vi "UpdateCameraSettings.vi"(10 "config":T1 {"QTrk Settings"."QI ROI Coverage" format="%_2g"; "QTrk Settings"."QI MinRadius" format="%.2f"; "QTrk Settings"."QI Angular sample density" format="%.3f"; "QTrk Settings"."QI Radial sample density" format="%.2f"; "QTrk Settings"."ZLUT Radial sample density" format="%.2f"; "QTrk Settings"."ZLUT MinRadius" format="%.2f"}, 11 "Main Camera Instance":T15) -> ()   [LabVIEW 2011]
uses:
  Main/Camera/CameraInstance.ctl
  Modules/CameraInterface/CameraInterface.ctl
  Modules/CameraInterface/CICloseType.ctl
  Modules/CameraInterface/CIGetSetGenericConfig.ctl
  Modules/CameraInterface/CIGrabType.ctl
  Modules/CameraInterface/CISettingsDlg.ctl
  Modules/CameraInterface/CIAdjustBeadPos.ctl
  Modules/CameraInterface/CISaveLoadSettings.ctl
  Main/Typedefs/MeasureConfigType.ctl
  Main/Typedefs/MeasureConfigOutputMode.ctl
  qtrk/QTrkLVBinding/QTrkSettings.ctl
  Main/Typedefs/TrackingConfigType.ctl
  qtrk/QTrkLVBinding/QTrkLocalizationType.ctl
  qtrk/QTrkLVBinding/QTrkZCommandType.ctl
  Main/ExperimentProgram/ExperimentProgramType.ctl
  Main/ExperimentProgram/ExProgCommandType.ctl
  Main/ExperimentProgram/ExProgCommandEnumType.ctl
  Main/Motors/MotorAxisEnum.ctl
  Main/Motors/MotorPosType.ctl
  Main/Typedefs/XYf.ctl
  Main/Motors/MotorPosFlagsType.ctl
  Main/Camera/GenericCameraConfigType.ctl
panel:
  # "(used for commands with string parameters)"
  # "-2: Use all devices\n-1: Use best device"
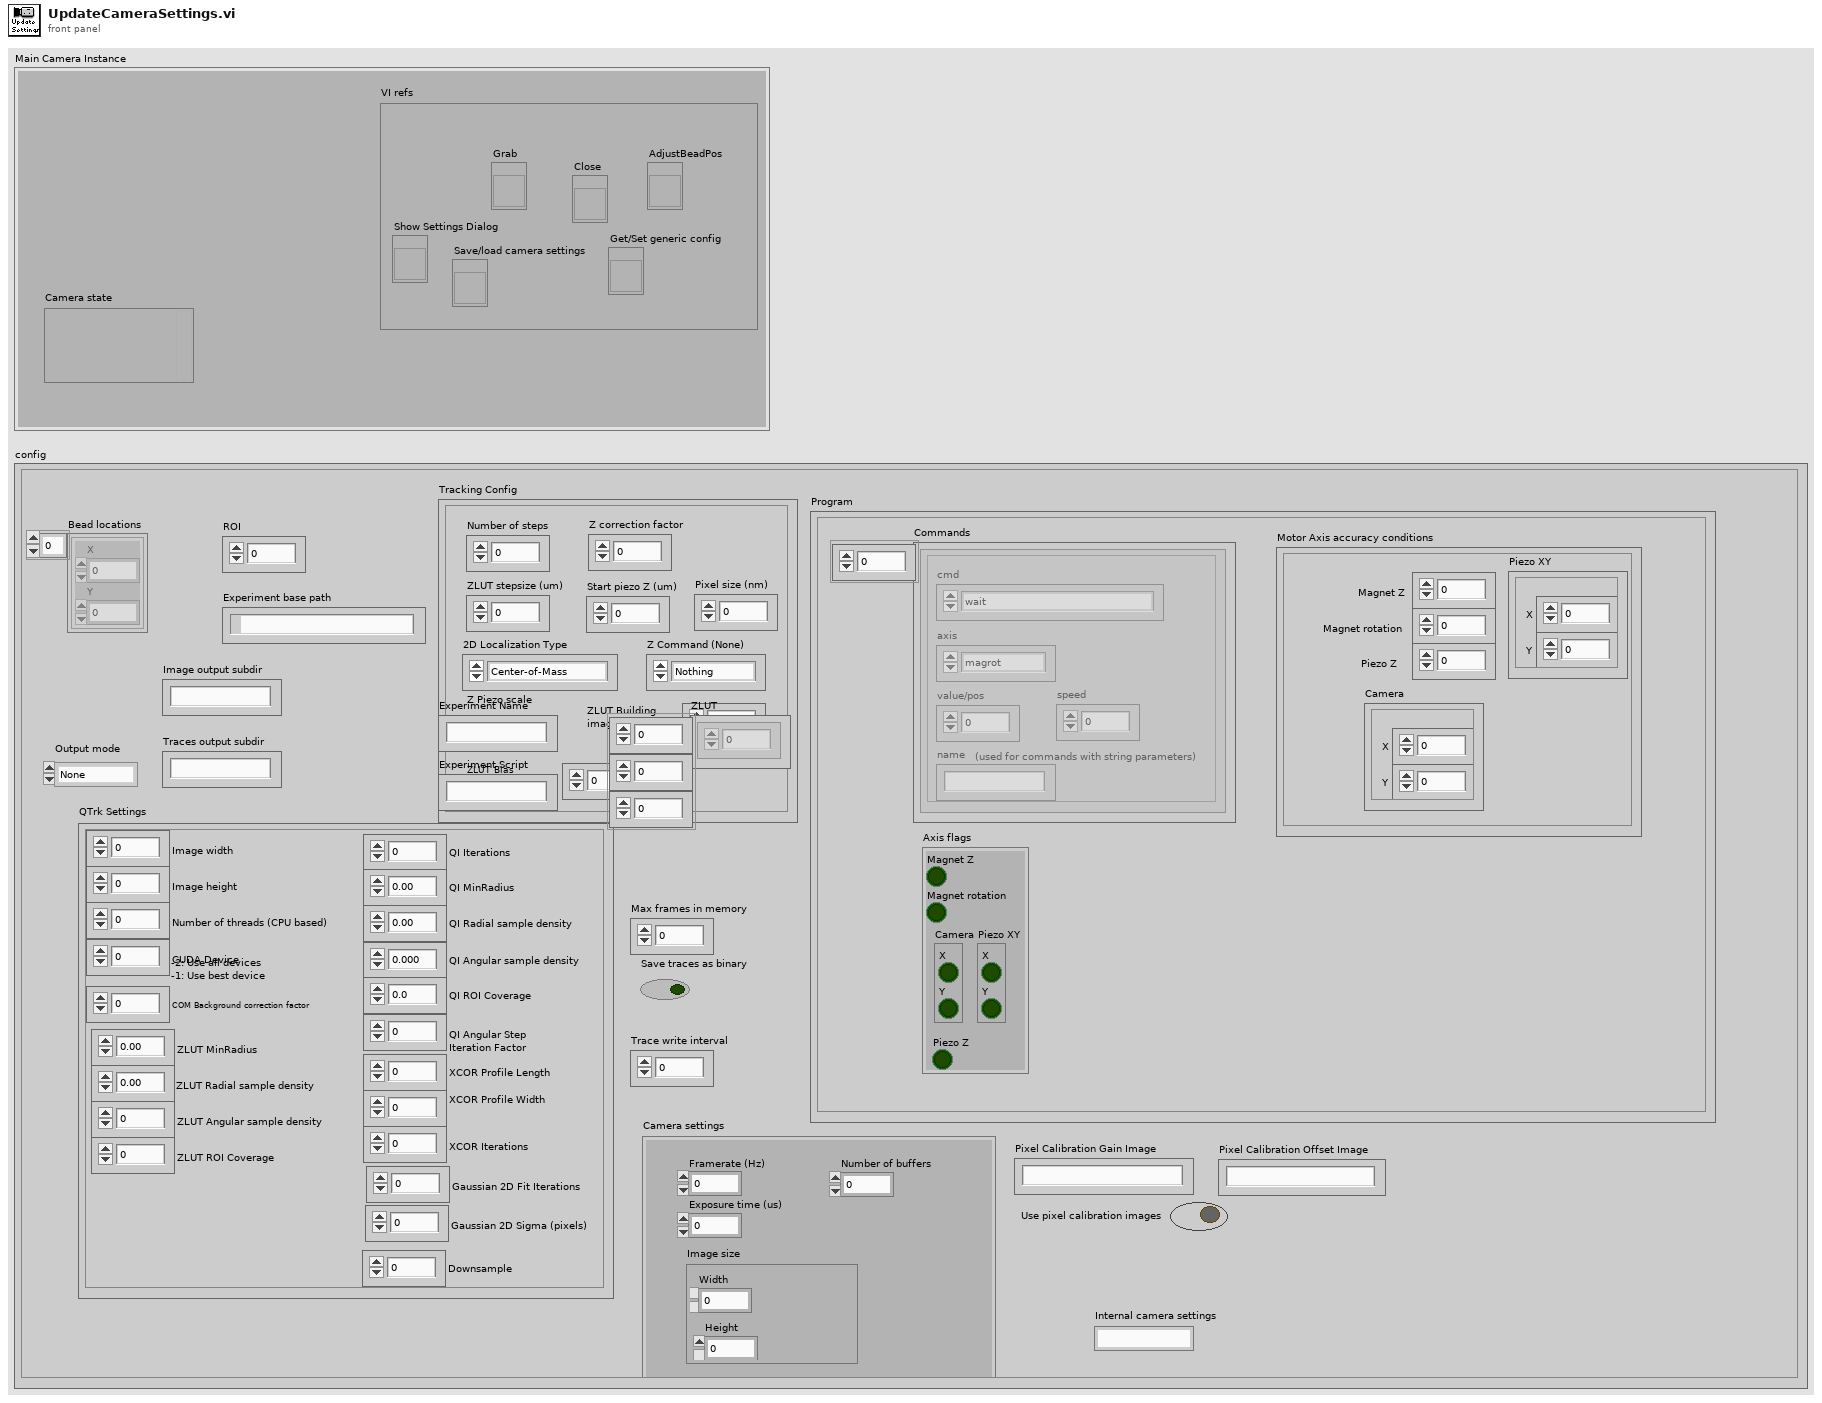
[diagram p1: front panel]
types:
  T1 = typedef "MeasureConfigType.ctl" = cluster{"Bead locations":cluster{"X":i32, "Y":i32}[], "ROI":i32, "Experiment base path":path, "Image output subdir":string, "Output mode":T2, "Traces output subdir":string, "QTrk Settings":T3, "Tracking Config":T4, "Experiment Name":string, "Program":T7, "ZLUT":sgl[][][], "Camera settings":T14, "Experiment Script":string, "Max frames in memory":i32, "Save traces as binary":bool, "Pixel Calibration Gain Image":string, "Pixel Calibration Offset Image":string, "Use pixel calibration images":bool, "Internal camera settings":string, "Trace write interval":i32}
  T2 = typedef "MeasureConfigOutputMode.ctl" = enum16{"None", "Track", "SaveImages"}
  T3 = typedef "QTrkSettings.ctl" = cluster{"Image width":i32, "Image height":i32, "Number of threads (CPU based)":i32, "CUDA Device":i32, "COM Background correction factor":sgl, "ZLUT MinRadius":sgl, "ZLUT Radial sample density":sgl, "ZLUT Angular sample density":sgl, "ZLUT ROI Coverage":sgl, "QI Iterations":i32, "QI MinRadius":sgl, "QI Radial sample density":sgl, "QI Angular sample density":sgl, "QI ROI Coverage":sgl, "QI Angular Step \nIteration Factor":sgl, "XCOR Profile Length":i32, "XCOR Profile Width":i32, "XCOR Iterations":i32, "Gaussian 2D Fit Iterations":i32, "Gaussian 2D Sigma (pixels)":sgl, "Downsample":i32}
  T4 = typedef "TrackingConfigType.ctl" = cluster{"Number of steps":i32, "ZLUT stepsize (um)":sgl, "Z correction factor":sgl, "Start piezo Z (um)":sgl, "Pixel size (nm)":sgl, "2D Localization Type":T5, "Z Command (None)":T6, "Z Piezo scale":bool, "ZLUT Building\nimages per frame":i32, "ZLUT Bias correction planes":i32}
  T5 = typedef "QTrkLocalizationType.ctl" = enum16{"Center-of-Mass", "1D Cross-Correlation", "Quadrant Interpolation", "Gaussian 2D MLE", "QI + ZLUTAlign", "ZLUTAlign", "QI + FourierLUT"}
  T6 = typedef "QTrkZCommandType.ctl" = enum16{"Nothing", "ComputeZ", "BuildRadialZLUT", "BuildImageZLUT", "RadialZLUT+ImageZLUT"}
  T7 = typedef "ExperimentProgramType.ctl" = cluster{"Commands":T8[], "Motor Axis accuracy conditions":T11, "Axis flags":T13}
  T8 = typedef "ExProgCommandType.ctl" = cluster{"cmd":T9, "axis":T10, "value/pos":dbl, "speed":dbl, "name":string}
  T9 = typedef "ExProgCommandEnumType.ctl" = enum16{"wait", "move", "event", "idle", "when", "section", "stop"}
  T10 = typedef "MotorAxisEnum.ctl" = enum16{"no axis", "magrot", "magpos", "px", "py", "pz", "camx", "camy"}
  T11 = typedef "MotorPosType.ctl" = cluster{"Magnet Z":dbl, "Magnet rotation":dbl, "Camera":T12, "Piezo XY":T12, "Piezo Z":dbl}
  T12 = typedef "XYf.ctl" = cluster{"X":sgl, "Y":sgl}
  T13 = typedef "MotorPosFlagsType.ctl" = cluster{"Magnet Z":bool, "Magnet rotation":bool, "Camera":cluster{"X":bool, "Y":bool}, "Piezo XY":cluster{"X":bool, "Y":bool}, "Piezo Z":bool}
  T14 = typedef "GenericCameraConfigType.ctl" = cluster{"Framerate (Hz)":i32, "Exposure time (us)":i32, "Image size":cluster{"Width":i32, "Height":i32}, "Number of buffers":i32}
  T15 = typedef "CameraInstance.ctl" = cluster{"VI refs":T16, "Camera state":variant}
  T16 = typedef "CameraInterface.ctl" = cluster{"Close":T17, "Get/Set generic config":T18, "Grab":T19, "Show Settings Dialog":T20, "AdjustBeadPos":T21, "Save/load camera settings":T22}
  T17 = typedef "CICloseType.ctl" = refnum<vi>
  T18 = typedef "CIGetSetGenericConfig.ctl" = refnum<vi>
  T19 = typedef "CIGrabType.ctl" = refnum<vi>
  T20 = typedef "CISettingsDlg.ctl" = refnum<vi>
  T21 = typedef "CIAdjustBeadPos.ctl" = refnum<vi>
  T22 = typedef "CISaveLoadSettings.ctl" = refnum<vi>
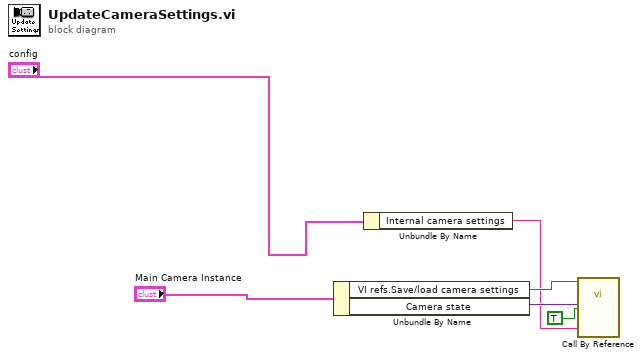
[diagram p0: block diagram]
diagram:
  n1 = Unbundle By Name("Main Camera Instance") -> ("VI refs.Save/load camera settings"=w3:T22, "Camera state"=w4:variant)
  n2 = Unbundle By Name("config") -> ("Internal camera settings"=w1:string)
  n3 = call-by-ref "?"(reference=w3, "Save?"=TRUE, "Serialized data"=w1, "Camera data"=w4) -> ()  [unwired: 8 in, 4 out]
